vi "set_pixel_dwell_time.vi"(8 "error in (no error)":errorcluster, 9 "number of sub-pattern points":dbl, 10 "pixel dwell time":dbl[unit], 11 "FPGAWrapperMH120124RAPS_PXI7813R in":refnum<class "FPGAWrapperMH120124RAPS_PXI7813R.lvclass">) -> (0 "error out":errorcluster, 3 "FPGAWrapperMH120124RAPS_PXI7813R out":refnum<class "FPGAWrapperMH120124RAPS_PXI7813R.lvclass">)   [LabVIEW 2010, in "FPGAWrapperMH120124RAPS_PXI7813R.lvclass"]
uses:
  FPGAWrapperMH120124RAPS_PXI7813R.lvclass
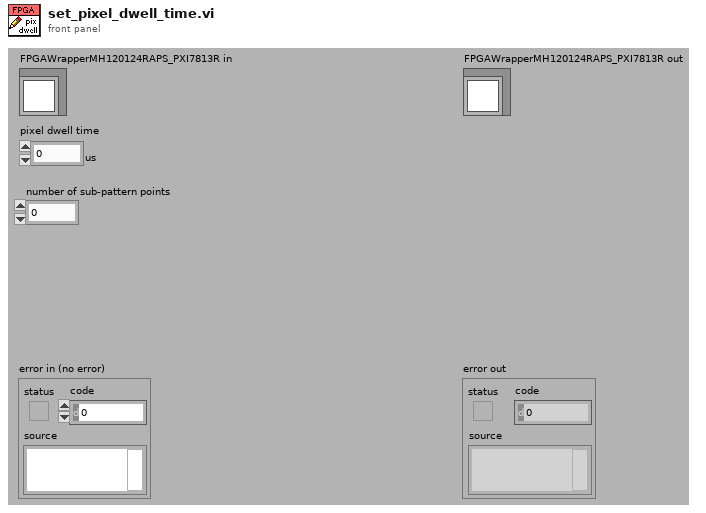
[diagram p1: front panel]
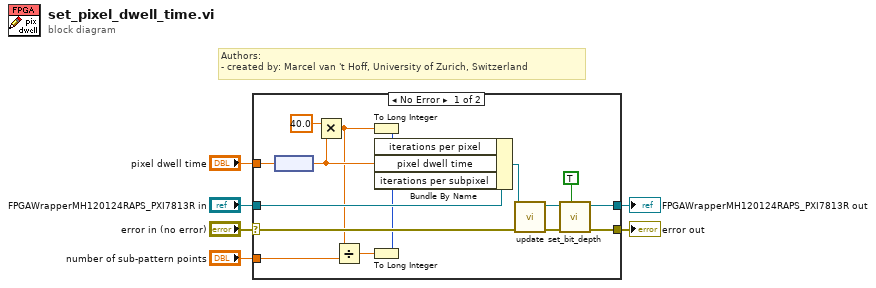
[diagram p0: block diagram]
diagram:
  # "Authors: \n- created by: Marcel van 't Hoff, University of Zurich, Switzerland"
  n1 = case shown="No Error" "error in (no error)" {
    selector: "error in (no error)" -> [w20 w23]
    tunnel: [w14 w23] -> w5
    tunnel: [w13 w24] -> w3
    tunnel: "FPGAWrapperMH120124RAPS_PXI7813R in" -> [w22 w24]
    tunnel: "pixel dwell time" -> [w21 _]
    tunnel: "number of sub-pattern points" -> [w10 _]
    frame No Error {
      n2 = node(w21) -> (w11:dbl)
      n3 = Multiply(x=40.0, y=w11) -> (x*y=w8:dbl)
      n4 = Divide(x=w8, y=w10) -> (x/y=w9:dbl)
      n5 = To Long Integer(number=w8) -> (32bit integer=w17:i32)
      n6 = To Long Integer(number=w9) -> (32bit integer=w7:i32)
      n7 = Bundle By Name(cluster=w22, "iterations per pixel"=w17, "pixel dwell time"=w11, "iterations per subpixel"=w7) -> (w19:refnum<class "FPGAWrapperMH120124RAPS_PXI7813R.lvclass">)
      n8 = call-dynamic "update.vi"("error in (no error)"=w20, "FPGAWrapperMH120124RAPS_PXI7813R in"=w19) -> ("error out"=w15:errorcluster, "FPGAWrapperMH120124RAPS_PXI7813R out"=w12:refnum<class "FPGAWrapperMH120124RAPS_PXI7813R.lvclass">)  [unwired: 8 in]
      n9 = call-dynamic "set_bit_depth.vi"("calculate by timing? (F)"=TRUE, "error in (no error)"=w15, "FPGAWrapperMH120124RAPS_PXI7813R in"=w12) -> ("error out"=w14:errorcluster, "FPGAWrapperMH120124RAPS_PXI7813R out"=w13:refnum<class "FPGAWrapperMH120124RAPS_PXI7813R.lvclass">)  [unwired: 7 in]
    }
    frame Error {
    }
  }
  "error out" <- w5
  "FPGAWrapperMH120124RAPS_PXI7813R out" <- w3
